vi "kalman transmit and receive state updates.vi"(7 "min photons to update":u32, 8 "update z":bool, 9 "update y":bool, 10 "update x":bool, 11 "3-axis PV tracking state":T2) -> (0 "Timed Out?":bool, 1 "measure ticks":u32, 2 "num kalmans queued":u16, 3 "3-axis PV tracking state out":T2, 4 "kalman to host":cluster{"Kalman State":T1, "Kalman Update":bool})   [LabVIEW 2010]
uses:
  kalman 3-axis state.ctl
  integrating single axis kalman state.ctl
  <vilib>/rvi/DataTransferAndStorage/Container/XNode/niFpgaContainer.xnode
  <vilib>/rvi/FXPMathLib/FxpMul/XNode/nifxpmath_Multiplier.xnode
  <vilib>/rvi/FXPMathLib/FxpMul/subVIs/nifxpmath_Mul_SimConfig.ctl
  <vilib>/fxp/LVFixedPointQuantizationPolicyTypeDef.ctl
  <vilib>/fxp/LVFixedPointOverflowPolicyTypeDef.ctl
  <vilib>/rvi/FIFO/Fifo_Resource/nirvififoEmulationSetSize.vi
  <vilib>/rvi/DataTransferAndStorage/Container/Common/niFpgaContainerGetUniqueNameForEmu.vi
  <vilib>/rvi/FXPMathLib/FxpMul/simVIs/DllFxpMulTemp_sub.vi
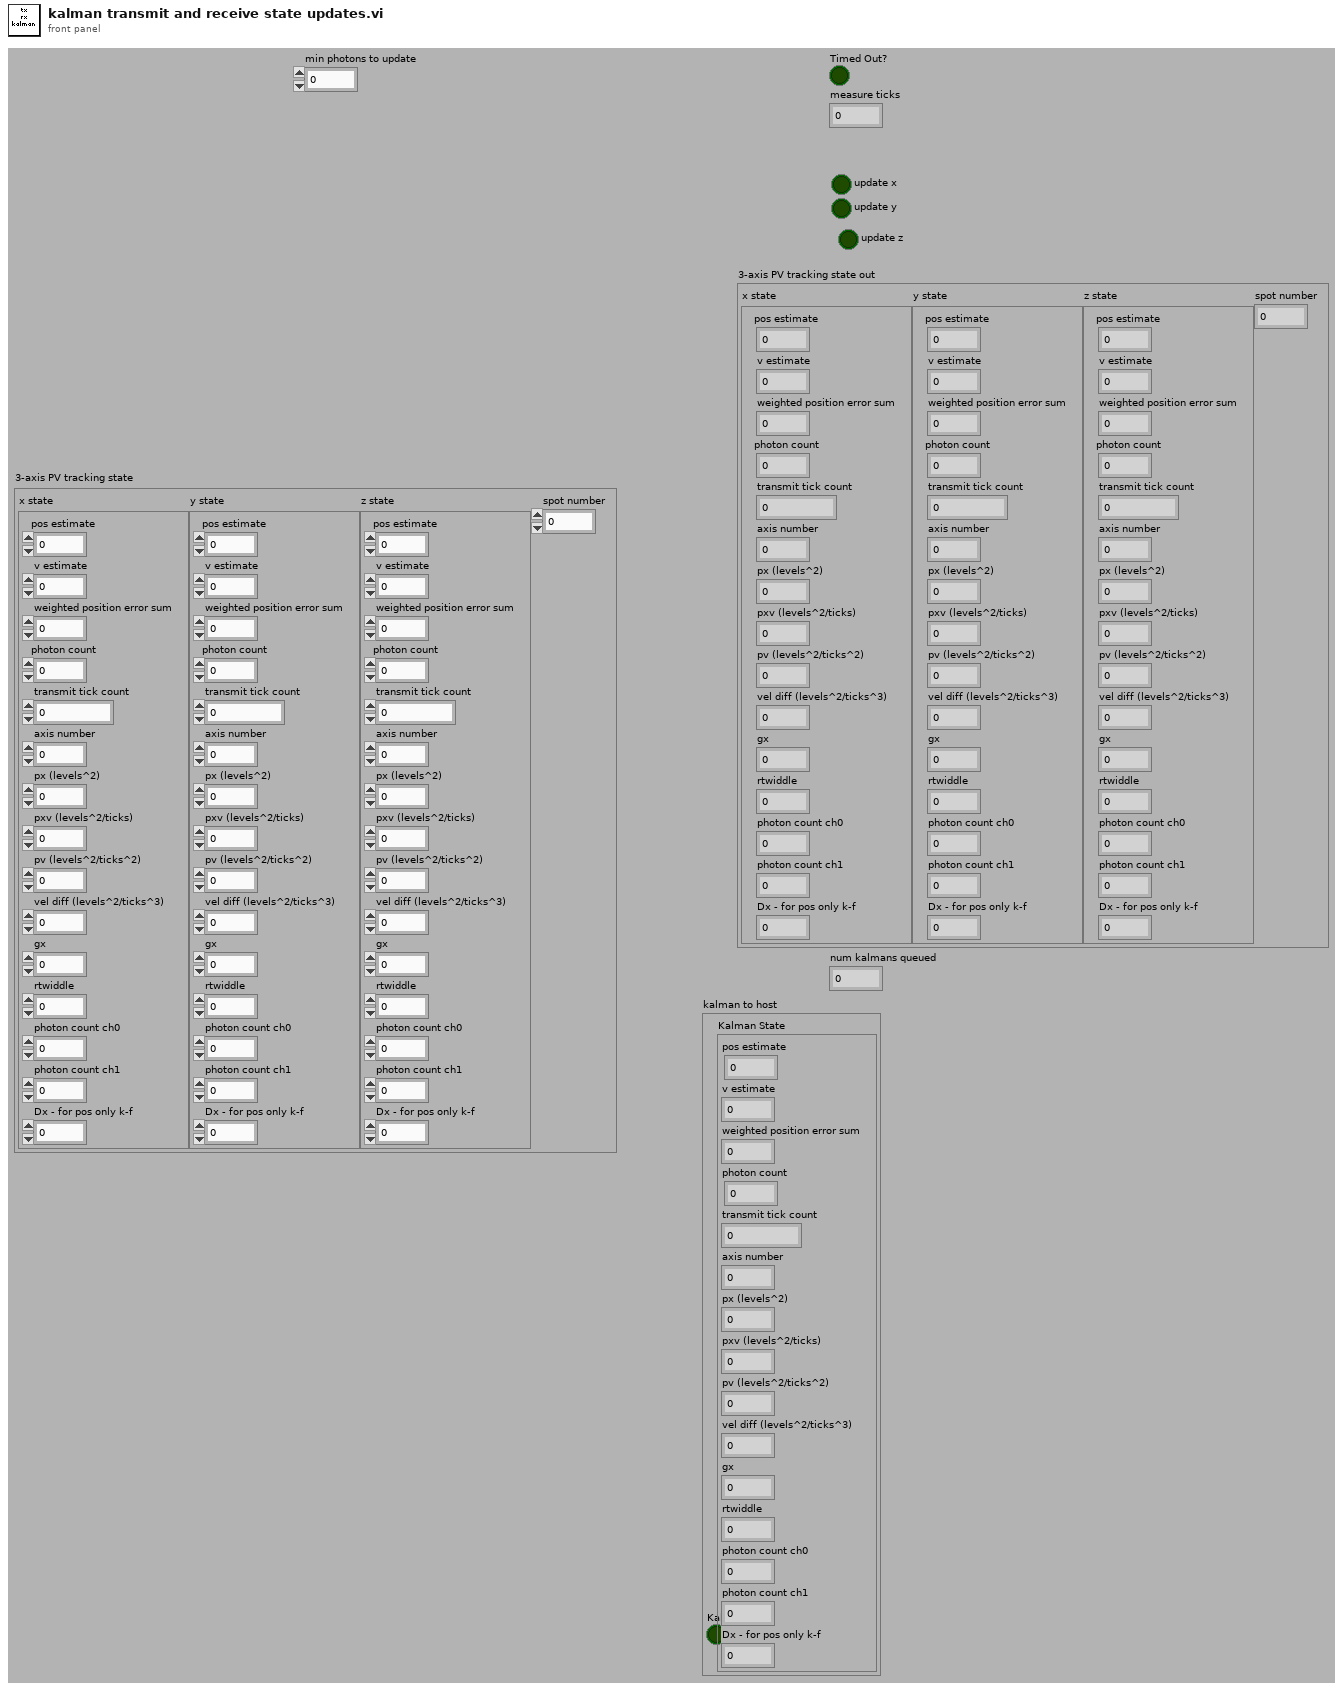
[diagram p1: front panel]
types:
  T1 = typedef "integrating single axis kalman state.ctl" = cluster{"pos estimate":fxp<+/-,32,16>, "v estimate":fxp<+/-,16,0>, "weighted position error sum":fxp<+/-,32,32>, "photon count":u32, "transmit tick count":u32, "axis number":u8, "px (levels^2)":fxp<+,32,19>, "pxv (levels^2/ticks)":fxp<+,32,2>, "pv (levels^2/ticks^2)":fxp<+,32,-14>, "vel diff (levels^2/ticks^3)":fxp<+,24,-22>, "gx":fxp<+,16,8>, "rtwiddle":fxp<+,16,26>, "photon count ch0":u32, "photon count ch1":u32, "Dx - for pos only k-f":fxp<+,32,19>}
  T2 = typedef "kalman 3-axis state.ctl" = cluster{"x state":T1, "y state":T1, "z state":T1, "spot number":u8}
  T3 = cluster{"pos estimate":fxp<+/-,32,16>, "v estimate":fxp<+/-,16,0>, "weighted position error sum":fxp<+/-,32,32>, "photon count":u32, "transmit tick count":u32, "axis number":u8, "px (levels^2)":fxp<+,32,19>, "pxv (levels^2/ticks)":fxp<+,32,2>, "pv (levels^2/ticks^2)":fxp<+,32,-14>, "vel diff (levels^2/ticks^3)":fxp<+,24,-22>, "gx":fxp<+,16,8>, "rtwiddle":fxp<+,16,26>, "photon count ch0":u32, "photon count ch1":u32, "Dx - for pos only k-f":fxp<+,32,19>}
  T4 = cluster{"Element":cluster{"pos estimate":fxp<+/-,32,16>, "v estimate":fxp<+/-,16,0>, "weighted position error sum":fxp<+/-,32,32>, "photon count":u32, "transmit tick count":u32, "axis number":u8, "px (levels^2)":fxp<+,32,19>, "pxv (levels^2/ticks)":fxp<+,32,2>, "pv (levels^2/ticks^2)":fxp<+,32,-14>, "vel diff (levels^2/ticks^3)":fxp<+,24,-22>, "gx":fxp<+,16,8>, "rtwiddle":fxp<+,16,26>, "photon count ch0":u32, "photon count ch1":u32, "Dx - for pos only k-f":fxp<+,32,19>}, bool}
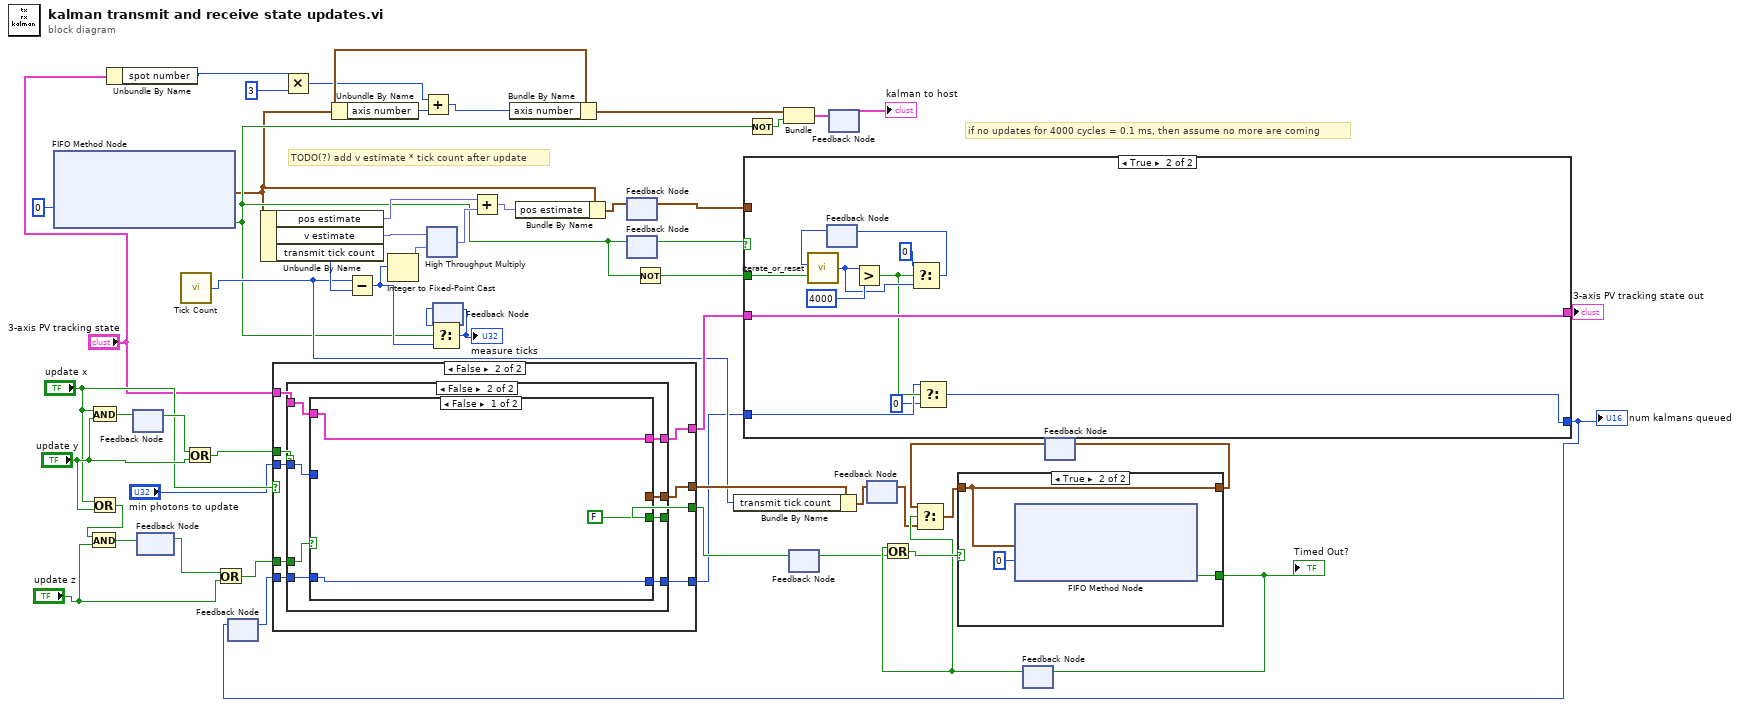
[diagram p0: block diagram]
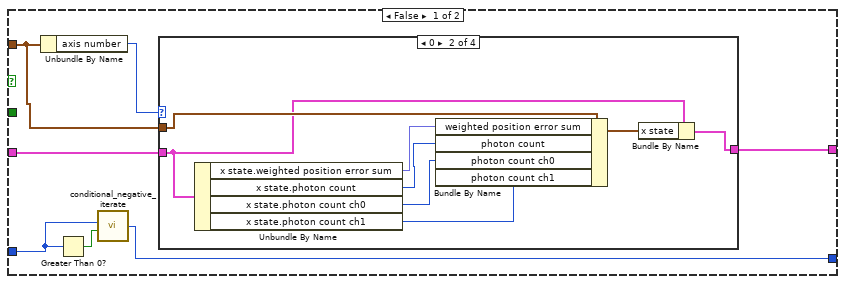
[diagram p2: hidden frame]
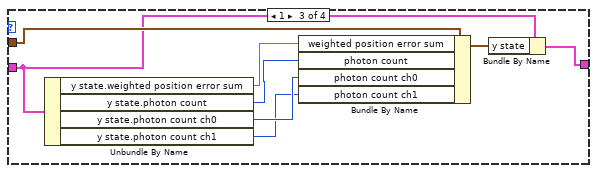
[diagram p4: hidden frame]
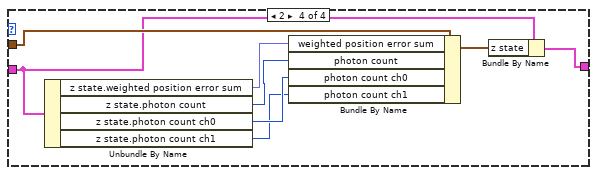
[diagram p5: hidden frame]
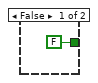
[diagram p6: hidden frame]
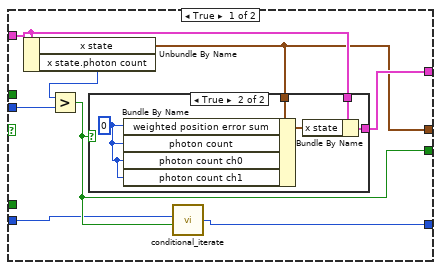
[diagram p7: hidden frame]
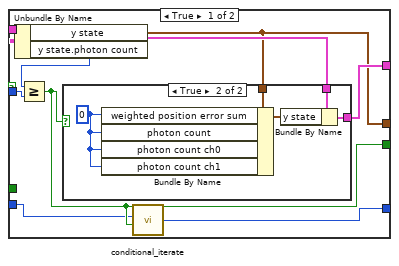
[diagram p9: hidden frame]
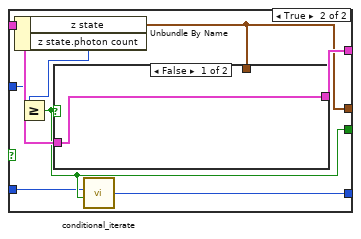
[diagram p11: hidden frame]
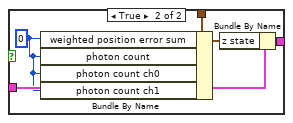
[diagram p12: hidden frame]
diagram:
  # "if no updates for 4000 cycles = 0.1 ms, then assume no more are coming"
  # "TODO(?) add v estimate * tick count after update"
  n1 = xnode ("FIFO Method Node")("Timeout"=0) -> ("Element"=w7:T3, "Timed Out?"=w10:bool)  [unwired: 1 in, 1 out]
  n2 = And(x="update x", y="update y") -> (x .and. y?=w54:bool)
  n3 = Or(x="update x", y="update y") -> (x .or. y?=w51:bool)
  n4 = And(x=w51, y="update z") -> (x .and. y?=w50:bool)
  n5 = Unbundle By Name("3-axis PV tracking state") -> ("spot number"=w1:u8)
  n6 = feedback-in #1(w54) -> ()
  n7 = feedback #1() -> (w53:bool)  [unwired: 1 in]
  n8 = feedback #2() -> (w49:bool)  [unwired: 1 in]
  n9 = feedback-in #2(w50) -> ()
  n10 = call "Tick Count"() -> ("Tick Count(Ticks)"=w29:u32)
  n11 = Or(x=w53, y="update y") -> (x .or. y?=w46:bool)
  n12 = Or(x=w49, y="update z") -> (x .or. y?=w45:bool)
  n13 = feedback #3() -> (w13:u16)  [unwired: 1 in]
  n14 = Unbundle By Name(w7) -> ("pos estimate"=w16:fxp<+/-,32,16>, "v estimate"=w21:fxp<+/-,16,0>, "transmit tick count"=w32:u32)
  n15 = case shown="False" "update x" {
    tunnel: "3-axis PV tracking state" -> [w62 w77]
    tunnel: [w61 w76] -> w36
    tunnel: [w60 w75] -> w43
    tunnel: [w57 w74] -> w44
    tunnel: w46 -> [_ w73]
    tunnel: w45 -> [_ w72]
    tunnel: "min photons to update" -> [w58 w71]
    tunnel: [w55 w70] -> w14
    tunnel: w13 -> [w56 w69]
    frame True {
      n16 = Unbundle By Name(w62) -> ("x state"=w60:T1, "x state.photon count"=w59:u32)
      n17 = Greater?(x=w59, y=w58) -> (0:w57:bool)
      n18 = case shown="True" w57 {
        tunnel: w62 -> [w63 w67]
        tunnel: [w63 w66] -> w61
        tunnel: w60 -> [_ w65]
        frame False {
        }
        frame True {
          w64 = i16 0
          n19 = Bundle By Name(cluster=w65, "weighted position error sum"=w64, "photon count"=w64, "photon count ch0"=w64, "photon count ch1"=w64) -> (w68:T1)
          n20 = Bundle By Name(cluster=w67, "x state"=w68) -> (w66:T2)
        }
      }
      n21 = call "conditional_iterate.vi"("iterate?"=w57, "number in"=w56) -> ("number out"=w55:u16)  [unwired: 4 in]
    }
    frame False {
      n22 = case shown="False" w73 {
        tunnel: w77 -> [w85 w99]
        tunnel: [w84 w98] -> w76
        tunnel: [w83 w97] -> w75
        tunnel: [w80 w96] -> w74
        tunnel: w72 -> [_ w95]
        tunnel: w71 -> [w82 w94]
        tunnel: [w78 w93] -> w70
        tunnel: w69 -> [w79 w92]
        frame True {
          n23 = Unbundle By Name(w85) -> ("y state"=w83:T1, "y state.photon count"=w81:u32)
          n24 = Greater Or Equal?(x=w81, y=w82) -> (x >= y?=w80:bool)
          n25 = case shown="True" w80 {
            tunnel: w85 -> [w86 w90]
            tunnel: [w86 w89] -> w84
            tunnel: w83 -> [_ w88]
            frame False {
            }
            frame True {
              w87 = i16 0
              n26 = Bundle By Name(cluster=w88, "weighted position error sum"=w87, "photon count"=w87, "photon count ch0"=w87, "photon count ch1"=w87) -> (w91:T1)
              n27 = Bundle By Name(cluster=w90, "y state"=w91) -> (w89:T2)
            }
          }
          n28 = call "conditional_iterate.vi"("iterate?"=w80, "number in"=w79) -> ("number out"=w78:u16)  [unwired: 4 in]
        }
        frame False {
          n29 = case shown="False" w95 {
            tunnel: w99 -> [w102 w110]
            tunnel: [w102 w109] -> w98
            tunnel: [_ w108] -> w97
            tunnel: [FALSE w105] -> w96
            tunnel: w94 -> [_ w107]
            tunnel: [w100 w104] -> w93
            tunnel: w92 -> [w100 w103]
            frame False {
            }
            frame True {
              n30 = Unbundle By Name(w110) -> ("z state"=w108:T1, "z state.photon count"=w106:u32)
              n31 = Greater Or Equal?(x=w106, y=w107) -> (x >= y?=w105:bool)
              n32 = case shown="False" w105 {
                tunnel: w110 -> [w111 w115]
                tunnel: [w111 w114] -> w109
                tunnel: w108 -> [_ w113]
                frame False {
                }
                frame True {
                  w112 = i16 0
                  n33 = Bundle By Name(cluster=w113, "weighted position error sum"=w112, "photon count"=w112, "photon count ch0"=w112, "photon count ch1"=w112) -> (w116:T1)
                  n34 = Bundle By Name(cluster=w115, "z state"=w116) -> (w114:T2)
                }
              }
              n35 = call "conditional_iterate.vi"("iterate?"=w105, "number in"=w103) -> ("number out"=w104:u16)  [unwired: 4 in]
            }
          }
        }
      }
    }
  }
  n36 = Multiply(x=w1, y=u8 3) -> (x*y=w4:u8)
  n37 = Unbundle By Name(w7) -> ("axis number"=w6:u8)
  n38 = Subtract(x=w29, y=w32) -> (x-y=w20:u32)
  n39 = Integer to Fixed-Point Cast(integer=w20) -> (fixed-point=w19:fxp<+,32,32>)  [unwired: 1 in]
  n40 = Add(x=w4, y=w6) -> (x+y=w3:u8)
  n41 = xnode "High Throughput Multiply"("x"=w21, "y"=w19) -> ("x*y"=w17:fxp<+/-,16,16>)
  n42 = feedback #4() -> (w25:u32)  [unwired: 1 in]
  n43 = Select(t=w25, s=w10, f=w20) -> (s? t:f=w26:u32)
  "measure ticks" <- w26
  n44 = feedback-in #4(w26) -> ()
  n45 = Add(x=w16, y=w17) -> (x+y=w18:fxp<+/-,32,16>)
  n46 = Bundle By Name(cluster=w7, "axis number"=w3) -> (w8:T3)
  n47 = Bundle By Name(cluster=w7, "pos estimate"=w18) -> (w31:T3)
  n48 = feedback-in #5(w31) -> ()
  n49 = feedback #5() -> (w24:T3)  [unwired: 1 in]
  n50 = feedback #6() -> (w11:bool)  [unwired: 1 in]
  n51 = feedback-in #6(w10) -> ()
  n52 = Not(x=w10) -> (.not. x?=w9:bool)
  n53 = Bundle By Name(cluster=w43, "transmit tick count"=w29) -> (w30:T1)
  n54 = case shown="True" w11 {
    tunnel: w24 -> [w120 _]
    tunnel: w36 -> [w122 w159]
    tunnel: [w121 w159] -> w35
    tunnel: w14 -> [w119 w151]
    tunnel: [w117 w149] -> w12
    tunnel: w9 -> [_ w158]
    frame False {
      n55 = Unbundle By Name(w120) -> ("axis number"=w123:u8)
      n56 = Greater Than 0?(x=w119) -> (x > 0?=w118:bool)
      n57 = call "conditional_negative_iterate.vi"("iterate?"=w118, "number in"=w119) -> ("number out"=w117:u16)  [unwired: 4 in]
      n58 = case shown="0" w123 {
        tunnel: w122 -> [w124 w129 w137 w145]
        tunnel: [w124 w127 w135 w143] -> w121
        tunnel: w120 -> [_ w132 w140 w148]
        frame Default {
        }
        frame 0 {
          n59 = Unbundle By Name(w129) -> ("x state.weighted position error sum"=w131:fxp<+/-,32,32>, "x state.photon count"=w130:u32, "x state.photon count ch0"=w126:u32, "x state.photon count ch1"=w125:u32)
          n60 = Bundle By Name(cluster=w132, "weighted position error sum"=w131, "photon count"=w130, "photon count ch0"=w126, "photon count ch1"=w125) -> (w128:T3)
          n61 = Bundle By Name(cluster=w129, "x state"=w128) -> (w127:T2)
        }
        frame 1 {
          n62 = Unbundle By Name(w137) -> ("y state.weighted position error sum"=w139:fxp<+/-,32,32>, "y state.photon count"=w138:u32, "y state.photon count ch0"=w134:u32, "y state.photon count ch1"=w133:u32)
          n63 = Bundle By Name(cluster=w140, "weighted position error sum"=w139, "photon count"=w138, "photon count ch0"=w134, "photon count ch1"=w133) -> (w136:T3)
          n64 = Bundle By Name(cluster=w137, "y state"=w136) -> (w135:T2)
        }
        frame 2 {
          n65 = Unbundle By Name(w145) -> ("z state.weighted position error sum"=w147:fxp<+/-,32,32>, "z state.photon count"=w146:u32, "z state.photon count ch0"=w142:u32, "z state.photon count ch1"=w141:u32)
          n66 = Bundle By Name(cluster=w148, "weighted position error sum"=w147, "photon count"=w146, "photon count ch0"=w142, "photon count ch1"=w141) -> (w144:T3)
          n67 = Bundle By Name(cluster=w145, "z state"=w144) -> (w143:T2)
        }
      }
    }
    frame True {
      n68 = feedback #7() -> (w157:u16)  [unwired: 1 in]
      n69 = call "iterate_or_reset.vi"("iterate?"=w158, "number in"=w157) -> ("number out"=w155:u16)  [unwired: 4 in]
      n70 = Greater?(x=w155, y=u16 4000) -> (0:w152:bool)
      n71 = Select(t=u16 0, s=w152, f=w155) -> (s? t:f=w153:u16)
      n72 = feedback-in #7(w153) -> ()
      n73 = Select(t=w151, s=w152, f=u16 0) -> (s? t:f=w149:u16)
    }
  }
  "3-axis PV tracking state out" <- w35
  "num kalmans queued" <- w12
  n74 = feedback-in #3(w12) -> ()
  n75 = Not(x=w10) -> (.not. x?=w22:bool)
  n76 = Bundle("Element"=w8, w22) -> (w23:T4)  [unwired: 1 in]
  n77 = feedback-in #8(w44) -> ()
  n78 = feedback #8() -> (w27:bool)  [unwired: 1 in]
  n79 = feedback-in #9(w23) -> ()
  n80 = feedback #9() -> (→"kalman to host":T4)  [unwired: 1 in]
  n81 = feedback-in #10(w30) -> ()
  n82 = feedback #10() -> (w28:T1)  [unwired: 1 in]
  n83 = feedback #11() -> (w39:bool)  [unwired: 1 in]
  n84 = Or(x=w39, y=w27) -> (x .or. y?=w40:bool)
  n85 = feedback #12() -> (w38:T1)  [unwired: 1 in]
  n86 = Select(t=w38, s=w39, f=w28) -> (s? t:f=w42:T1)
  n87 = case shown="True" w40 {
    tunnel: w42 -> [_ w161]
    tunnel: [FALSE ("Timed Out?") w162] -> w41
    tunnel: [_ w161] -> w33
    frame False {
    }
    frame True {
      n88 = xnode ("FIFO Method Node")("Element"=w161, "Timeout"=0) -> ("Timed Out?"=w162:bool)  [unwired: 1 in, 1 out]
    }
  }
  "Timed Out?" <- w41
  n89 = feedback-in #11(w41) -> ()
  n90 = feedback-in #12(w33) -> ()
